vi "channel post scan properties.vi"(10 "scan_desc":T1, 11 "chav":T2[](array[typedef])) -> (3 "Computed channel properties":cluster{"Split index":dbl, "sample_rate":dbl}[](array[cluster]))   [LabVIEW 2021]
doc: "Helper to compute post scan properties."
uses:
  <userlib>/libad4/controls/ad scan cha desc.ctl
  <userlib>/libad4/controls/ad scan desc.ctl
  <userlib>/libad4/libad4.lvlib
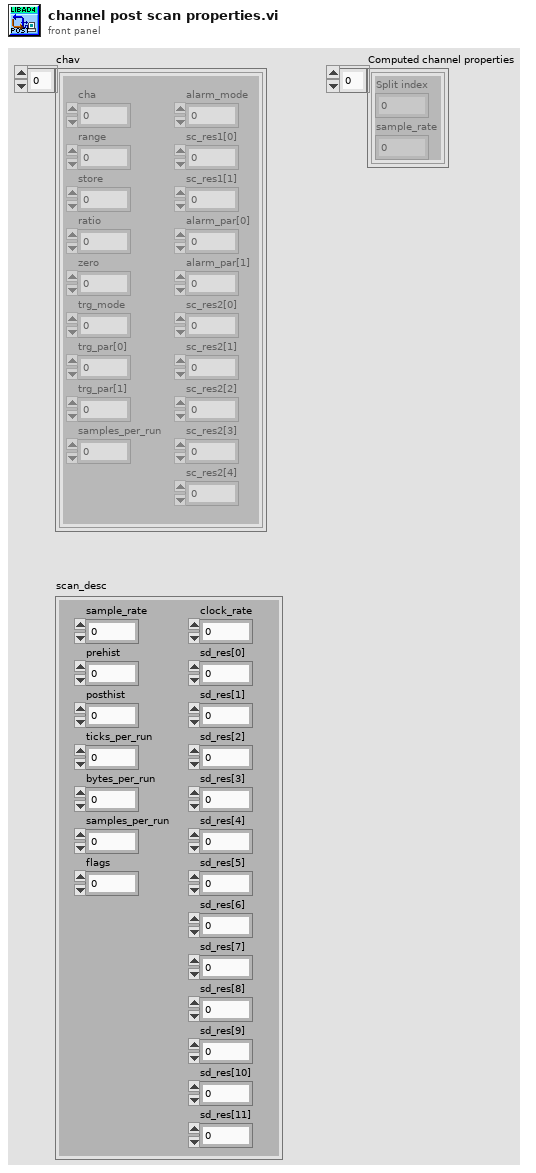
[diagram p1: front panel]
types:
  T1 = typedef "libad4.lvlib/ad scan desc.ctl" = cluster{"sample_rate":dbl, "clock_rate":dbl, "prehist":u64, "posthist":u64, "ticks_per_run":u32, "bytes_per_run":u32, "samples_per_run":u32, "flags":u32, "sd_res[0]":u32, "sd_res[1]":u32, "sd_res[2]":u32, "sd_res[3]":u32, "sd_res[4]":u32, "sd_res[5]":u32, "sd_res[6]":u32, "sd_res[7]":u32, "sd_res[8]":u32, "sd_res[9]":u32, "sd_res[10]":u32, "sd_res[11]":u32}
  T2 = typedef "libad4.lvlib/ad scan cha desc.ctl" = cluster{"cha":i32, "range":i32, "store":i32, "ratio":i32, "zero":u32, "trg_mode":u8, "alarm_mode":u8, "sc_res1[0]":u8, "sc_res1[1]":u8, "trg_par[0]":u32, "trg_par[1]":u32, "samples_per_run":i32, "alarm_par[0]":u32, "alarm_par[1]":u32, "sc_res2[0]":u32, "sc_res2[1]":u32, "sc_res2[2]":u32, "sc_res2[3]":u32, "sc_res2[4]":u32}
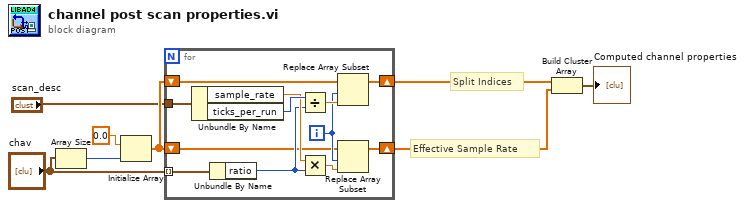
[diagram p0: block diagram]
diagram:
  # "Effective Sample Rate"
  # "Split Indices"
  n1 = Array Size(array="chav") -> (size(s)=w7:i32)
  n2 = Initialize Array(0.0 ("element"), w7) -> (w5:dbl[])
  n3 = for {
    tunnel: "chav" -> [w20] mode=indexing
    tunnel: "scan_desc" -> [w19]
    shift-right: [w16] -> w4
    shift-left: w5 -> [w15]
    shift-right: [w10] -> w3
    shift-left: w5 -> [w11]
    i -> [w12]
    n4 = Unbundle By Name(w19) -> ("sample_rate"=w14:dbl, "ticks_per_run"=w18:u32)
    n5 = Unbundle By Name(w20) -> ("ratio"=w13:i32)
    n6 = Divide(x=w18, y=w13) -> (x/y=w17:dbl)
    n7 = Multiply(x=w14, y=w13) -> (x*y=w9:dbl)
    n8 = Replace Array Subset(array=w15, new element=w17, index=w12) -> (w16:dbl[])
    n9 = Replace Array Subset(array=w11, new element=w9, index=w12) -> (w10:dbl[])
  }
  n10 = Build Cluster Array(w4, w3) -> (→"Computed channel properties":cluster{"element":dbl, "element":dbl}[])
